vi "DMAC U64 to DMAC U8.vi"(5 "DMAC U64":u64 format="%012x") -> (2 "DestinationMACAddress":u8[](array[numeric])=[3, 0, 94, 160, 3, 233] format="%02x")   [LabVIEW 2021, in "Networking_CIF_U.lvlib"]
uses:
  Networking_CIF_U.lvlib
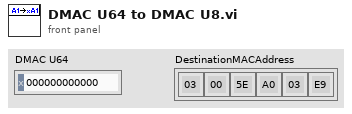
[diagram p1: front panel]
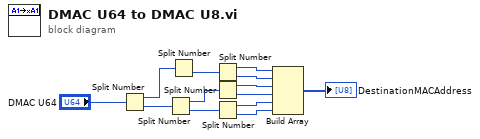
[diagram p0: block diagram]
diagram:
  n1 = Split Number(x="DMAC U64") -> (hi(x)=w9:u32, lo(x)=w12:u32)
  n2 = Split Number(x=w12) -> (hi(x)=w10:u16, lo(x)=w11:u16)
  n3 = Split Number(x=w9) -> (lo(x)=w8:u16)  [unwired: 1 out]
  n4 = Split Number(x=w8) -> (hi(x)=w7:u8, lo(x)=w6:u8)
  n5 = Split Number(x=w10) -> (hi(x)=w5:u8, lo(x)=w4:u8)
  n6 = Split Number(x=w11) -> (hi(x)=w3:u8, lo(x)=w2:u8)
  n7 = Build Array(w7, w6, w5, w4, w3, w2) -> (→"DestinationMACAddress":u8[])
